vi "Periodic Tasks.vi"(8 "error in":errorcluster) -> ()   [LabVIEW 2017]
doc: "This VI runs in parallel to other tasks. It can contain as many user-defined periodic loops as you need. These can carry out PID or other sorts of timed response."
uses:
  <vilib>/Rock Robotics/WPI/Solenoid/WPI_SolenoidValue.ctl
  <vilib>/Rock Robotics/Network Tables/NT Write Number.vi
  <vilib>/Rock Robotics/WPI/Utilities/WPI_GetSetVariantRefNum.vi
  Robot Global Data.vi
  <vilib>/Rock Robotics/WPI/RobotDrive/WPI_RobotDriveMecanumDrive_Cartesian.vi
  <vilib>/Rock Robotics/Network Tables/NT Write Numeric Array.vi
  <vilib>/Rock Robotics/Network Tables/NT Write Boolean.vi
  <vilib>/Rock Robotics/WPI/Solenoid/WPI_SolenoidSetEnum.vi
  <vilib>/Rock Robotics/WPI/ThirdParty/Sensors/ADIS16448 IMU/ADIS16448_IMU.lvlib
  <vilib>/addons/control/pid/NI_PID_pid.lvlib
  <vilib>/addons/control/pid/pid.llb/PID (DBL).vi
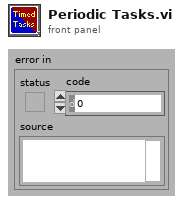
[diagram p1: front panel]
types:
  T1 = typedef "WPI_RobotDriveDevRef.ctl" = cluster{"DevStatus":errorcluster, "Motors[]":T2[], "Square Inputs":bool, "Max Output":dbl}
  T2 = typedef "WPI_MotorControlDeviceRef.ctl" = cluster{"DeviceStatus":errorcluster, "Type":T3, "PWM":cluster{"PWM Channel":T4, "DeadBand":T5}, "CAN":cluster{"Device Number":u8, "SetOutput VI Ref":variant, "GetOutput VI Ref":variant, "Enable VI Ref":variant, "Disable VI Ref":variant, "Data":variant}, "Invert":bool, "DIO PWM":cluster{"PWM \"Enable\" Channel":T4, "DIOChannel":T6, "PWM Rate":dbl}}
  T3 = typedef "WPI_MotorControlType.ctl" = enum16{"PWM", "CAN", "DIO PWM"}
  T4 = typedef "FPGA_DIOPWMChannel.ctl" = enum8{"PWM 0", "PWM 1", "PWM 2", "PWM 3", "PWM 4", "PWM 5", "PWM 6", "PWM 7", "PWM 8", "PWM 9", "PWM MXP 0", "PWM MXP 1", "PWM MXP 2", "PWM MXP 3", "PWM MXP 4", "PWM MXP 5", "PWM MXP 6", "PWM MXP 7", "PWM MXP 8", "PWM MXP 9", "Invalid"}
  T5 = typedef "WPI_PWMDeadband.ctl" = cluster{"Name":string, "maxPositivePwm":i32, "minPositivePwm":i32, "centerPwm":i32, "maxNegativePwm":i32, "minNegativePwm":i32, "angularRange":u16}
  T6 = typedef "FPGA_DIOChannel.ctl" = enum8{"DIO 0", "DIO 1", "DIO 2", "DIO 3", "DIO 4", "DIO 5", "DIO 6", "DIO 7", "DIO 8", "DIO 9", "DIO MXP 0", "DIO MXP 1", "DIO MXP 2", "DIO MXP 3", "DIO MXP 4", "DIO MXP 5", "DIO MXP 6", "DIO MXP 7", "DIO MXP 8", "DIO MXP 9", "DIO MXP 10", "DIO MXP 11", "DIO MXP 12", "DIO MXP 13", "DIO MXP 14", "DIO MXP 15", "SPI Port CS1", "SPI Port CS2", "SPI Port CS3", "SPI Port MISO", "SPI Port MOSI", "Invalid"}
  T7 = typedef "WPI_SolenoidDevRef.ctl" = cluster{"DevStatus":errorcluster, "Pneumatics Control Module":u8, "Forward Solenoid Channel":T8, "Reverse Solenoid Channel":T8}
  T8 = typedef "WPI_SolenoidChannel.ctl" = enum8{"Solenoid 0", "Solenoid 1", "Solenoid 2", "Solenoid 3", "Solenoid 4", "Solenoid 5", "Solenoid 6", "Solenoid 7", "Invalid"}
  T9 = typedef "ADIS16448_IMU.lvlib/ADI_IMU_ADIS16448_IMUDevRef.ctl" = cluster{"DevStatus":errorcluster, "Handle":i32, "SPI Bus":T10, "Device Found":bool, "Device Ready":bool, "Yaw Axis":enum16{"X", "Y", "Z"}, "AHRS Algorithm":enum16{"Complementary", "Madgwick"}, "Serial":u16, "Lot ID 2":u16, "Lot ID 1":u16, "Bytes Per Sample":u16, "Calibrate On Open?":bool}
  T10 = typedef "spi_bus.ctl" = enum16{"SPI On-Board, CS0", "SPI On-Board, CS1", "SPI On-Board, CS2", "SPI On-Board, CS3", "SPI MXP", "Invalid"}
  T11 = typedef "WPI_CompressorDevRef.ctl" = cluster{"DevStatus":errorcluster, "Pneumatics Control Module":u8}
  T12 = typedef "WPI_SolenoidValue.ctl" = enum16{"Off", "On", "Forward", "Reverse"}
  T13 = cluster{"proportional gain (Kc)":dbl, "integral time (Ti, min)":dbl, "derivative time (Td, min)":dbl}
  T14 = cluster{"X Angle":dbl, "Y Angle":dbl, "Z Angle":dbl}
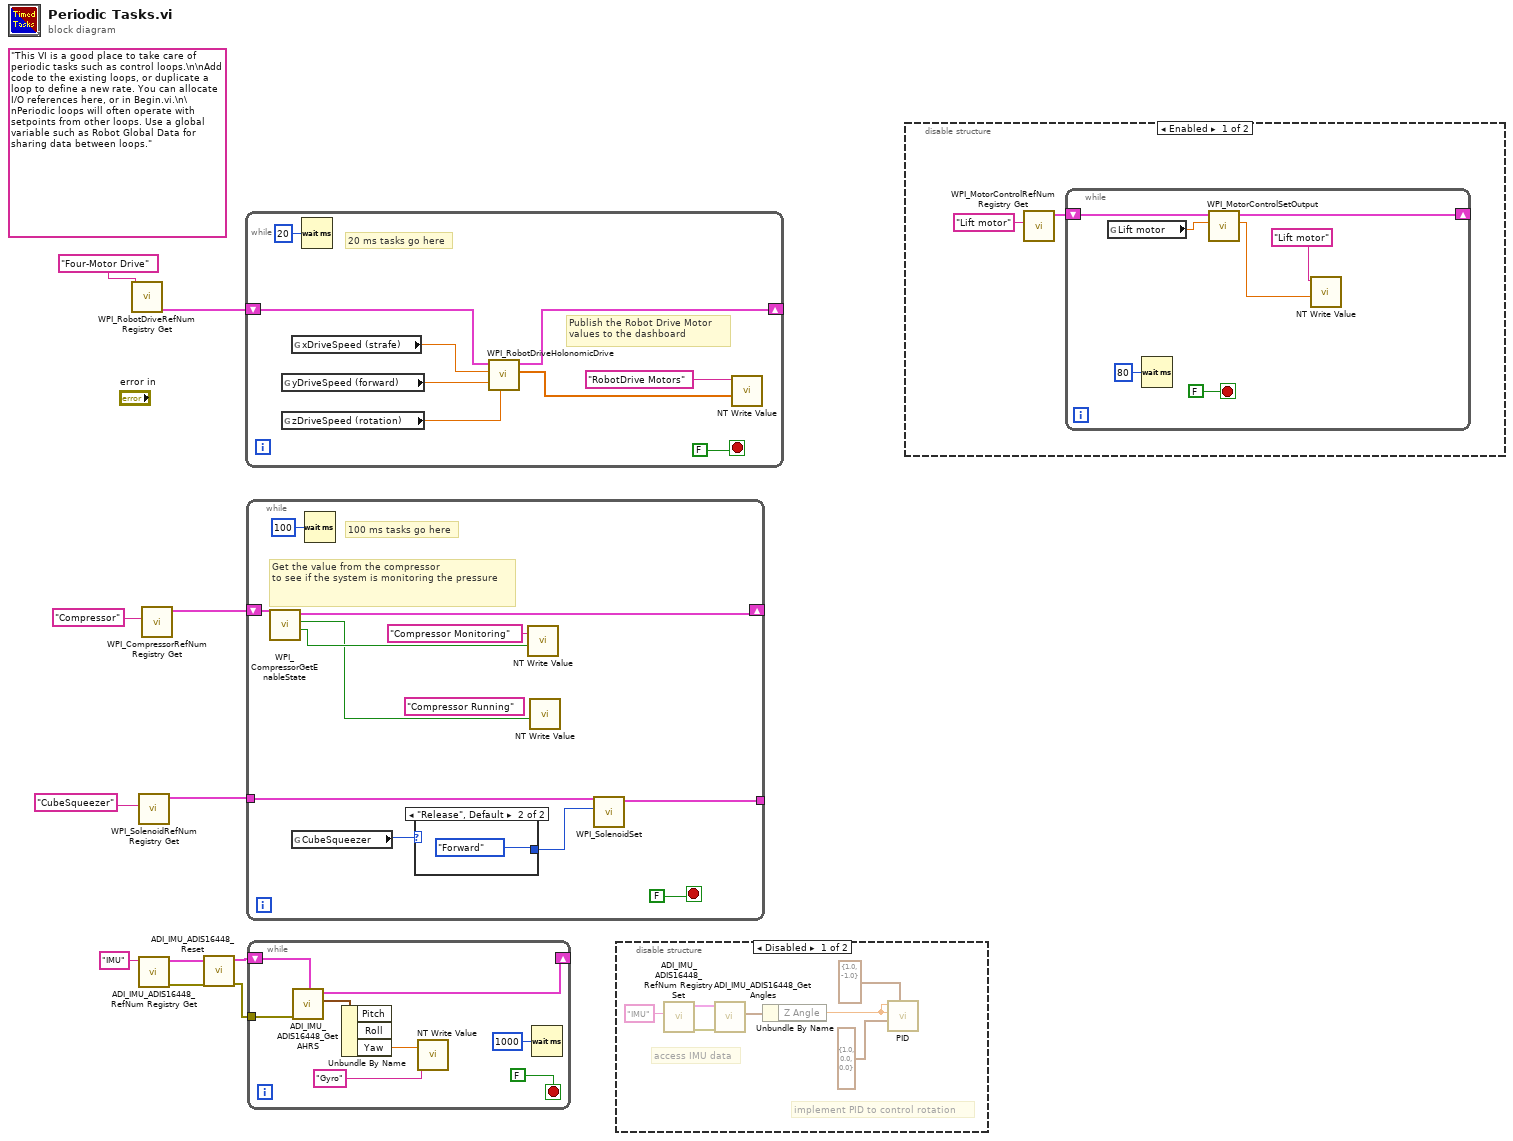
[diagram p0: block diagram]
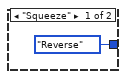
[diagram p4: hidden frame]
diagram:
  (unwired) "This VI is a good place to take care of periodic tasks such as control loops.\n\nAdd code to the existing loops, or duplicate a loop to define a new rate. You can allocate I/O references here, or in Begin.vi.\n\nPeriodic loops will often operate with setpoints from other loops. Use a global variable such as Robot Global Data for sharing data between loops."
  n1 = call <vilib>:"WPI_RobotDriveRefNum Registry Get.vi"("refnum name"="Four-Motor Drive") -> ("RobotDriveDevRef"=w5:T1)  [unwired: 1 in, 9 out]
  n2 = call <vilib>:"WPI_SolenoidRefNum Registry Get.vi"("refnum name"="CubeSqueezer") -> ("SolenoidDevRef"=w3:T7)  [unwired: 9 in, 1 out]
  n3 = call <vilib>:"ADI_IMU_ADIS16448_RefNum Registry Get.vi"("refnum name"="IMU") -> ("error out"=w9:errorcluster, "ADI IMU DevRef"=w10:T9)  [unwired: 9 in]
  n4 = call <vilib>:"WPI_CompressorRefNum Registry Get.vi"("refnum name"="Compressor") -> ("CompressorDevRef"=w2:T11)  [unwired: 9 in, 1 out]
  n5 = call <vilib>:"ADI_IMU_ADIS16448_Reset.vi"("error in"=w9, "ADI IMU DevRef"=w10) -> ("error out"=w8:errorcluster, "ADI IMU DevRef Out"=w11:T9)  [unwired: 8 in]
  n6 = while {
    shift-right: [w15] -> _
    shift-left: w5 -> [w16]
    stop <- FALSE stop-if-true
    # "Publish the Robot Drive Motor\nvalues to the dashboard"
    # "20 ms tasks go here"
    n7 = global read "Robot Global Data.vi" "yDriveSpeed (forward)"() -> (w13:dbl)
    n8 = global read "Robot Global Data.vi" "zDriveSpeed (rotation)"() -> (w12:dbl)
    n9 = global read "Robot Global Data.vi" "xDriveSpeed (strafe)"() -> (w14:dbl)
    n10 = Wait (ms)(milliseconds to wait=u32 20) -> ()  [unwired: 1 out]
    n11 = call-poly <vilib>:"WPI_RobotDriveHolonomicDrive.vi"("Rotation"=w12, "Y"=w13, "X"=w14, "RobotDriveDevRef"=w16) -> ("Motor Values"=w18:dbl[], "RobotDriveDevRef"=w15:T1)  [unwired: 5 in, 1 out]
    n12 = call-poly <vilib>:"NT Write Value.vi"("Numeric Array"=w18, "Name"="RobotDrive Motors") -> ()  [unwired: 9 in, 1 out]
  }
  n13 = while {
    shift-right: [w28] -> _
    shift-left: w2 -> [w29]
    tunnel: w3 -> [w27]
    tunnel: [w26] -> _
    stop <- FALSE stop-if-true
    (unwired) "Compressor Running" ("Name")
    # "Get the value from the compressor \nto see if the system is monitoring the pressure"
    # "100 ms tasks go here"
    n14 = call <vilib>:"WPI_CompressorGetEnableState.vi"("CompressorDevRef"=w29) -> ("Compressor Running"=w22:bool, "Enabled"=w21:bool, "CompressorDevRef"=w28:T11)  [unwired: 1 in, 7 out]
    n15 = global read "Robot Global Data.vi" "CubeSqueezer"() -> (w24:enum16{"Squeeze", "Release"})
    n16 = Wait (ms)(milliseconds to wait=u32 100) -> ()  [unwired: 1 out]
    n17 = case shown="\"Release\", Default" w24 {
      tunnel: [WPI_SolenoidValue."Reverse" ("Value") WPI_SolenoidValue."Forward" ("Value")] -> w25
      frame "Squeeze" {
      }
      frame "Release", Default {
      }
    }
    n18 = call-poly <vilib>:"NT Write Value.vi"("Boolean"=w22, "Name"="Compressor Monitoring") -> ()  [unwired: 9 in, 1 out]
    n19 = call-poly <vilib>:"NT Write Value.vi"("Boolean"=w21) -> ()  [unwired: 10 in, 1 out]
    n20 = call-poly <vilib>:"WPI_SolenoidSet.vi"("Value"=w25, "SolenoidDevRef"=w27) -> ("SolenoidDevRef"=w26:T7)  [unwired: 8 in, 1 out]
  }
  n21 = while {
    shift-right: [w40] -> _
    shift-left: w11 -> [w41]
    tunnel: w8 -> [w34]
    stop <- FALSE stop-if-true
    n22 = call <vilib>:"ADI_IMU_ADIS16448_Get AHRS.vi"("error in"=w34, "ADI IMU DevRef"=w41) -> ("IMU AHRS Out"=w37:cluster{"Pitch":dbl, "Roll":dbl, "Yaw":dbl}, "ADI IMU DevRef Out"=w40:T9)  [unwired: 6 in, 2 out]
    n23 = Unbundle By Name(w37) -> ("Yaw"=w36:dbl)  [unwired: 2 out]
    n24 = call-poly <vilib>:"NT Write Value.vi"("Numeric"=w36, "Name"="Gyro") -> ()  [unwired: 9 in, 1 out]
    n25 = Wait (ms)(milliseconds to wait=u32 1000) -> ()  [unwired: 1 out]
  }
  n26 = disable-structure shown="Disabled" {
    frame Disabled {
      # "implement PID to control rotation"
      # "access IMU data"
      n27 = call <vilib>:"ADI_IMU_ADIS16448_RefNum Registry Set.vi"("refnum name"="IMU") -> ("error out"=w47:errorcluster, "ADI IMU DevRef"=w46:T9)  [unwired: 9 in]
      n28 = call <vilib>:"ADI_IMU_ADIS16448_Get Angles.vi"("error in"=w47, "ADI IMU DevRef"=w46) -> ("IMU Angles Out"=w45:T14)  [unwired: 6 in, 3 out]
      n29 = Unbundle By Name(w45) -> ("Z Angle"=w44:dbl)
      n30 = call-poly <vilib>:"PID.vi"("output range"=cluster{"output high":dbl, "output low":dbl} {"output high"=1.0, "output low"=-1.0}, "PID gains"=T13 {"proportional gain (Kc)"=1.0, "integral time (Ti, min)"=0.0, "derivative time (Td, min)"=0.0}, "process variable"=w44, "setpoint"=w44) -> ()  [unwired: 6 in, 2 out]
    }
    frame Enabled {
    }
  }
  n31 = disable-structure shown="Enabled" {
    frame Enabled {
      n32 = call <vilib>:"WPI_MotorControlRefNum Registry Get.vi"("refnum name"="Lift motor") -> ("MotorControlDevRef"=w50:T2)  [unwired: 9 in, 1 out]
      n33 = while {
        shift-right: [w57] -> _
        shift-left: w50 -> [w54]
        stop <- FALSE stop-if-true
        n34 = global read "Robot Global Data.vi" "Lift motor"() -> (w53:dbl)
        n35 = Wait (ms)(milliseconds to wait=u32 80) -> ()  [unwired: 1 out]
        n36 = call <vilib>:"WPI_MotorControlSetOutput.vi"("Output"=w53, "MotorControlDevRef"=w54) -> ("Motor Output"=w52:dbl, "MotorControlDevRef"=w57:T2)  [unwired: 7 in, 1 out]
        n37 = call-poly <vilib>:"NT Write Value.vi"("Numeric"=w52, "Name"="Lift motor") -> ()  [unwired: 9 in, 1 out]
      }
    }
    frame Disabled {
    }
  }
